vi "SizeGraphPanel.vi"(8 "ErrorIn(No Error)":errorcluster caption="entrée d'erreur (pas d'erreur)", 9 "Width Divider":i32, 10 "Height Divider":i32, 11 "PanRef":refnum<vi>) -> (0 "sortie d'erreur":errorcluster, 2 "Position":T1, 3 "cluster de sortie":T2 caption="Taille")   [LabVIEW 2010]
uses:
  <vilib>/Utility/miscctls.llb/LVBoundsTypeDef.ctl
  <vilib>/Utility/miscctls.llb/LVPositionTypeDef.ctl
  System.Windows.Forms
  System.Drawing
  <vilib>/Utility/miscctls.llb/LVPointTypeDef.ctl
panel:
  out "UpdtHorizLim":bool
  out "UpdtVertLim":bool
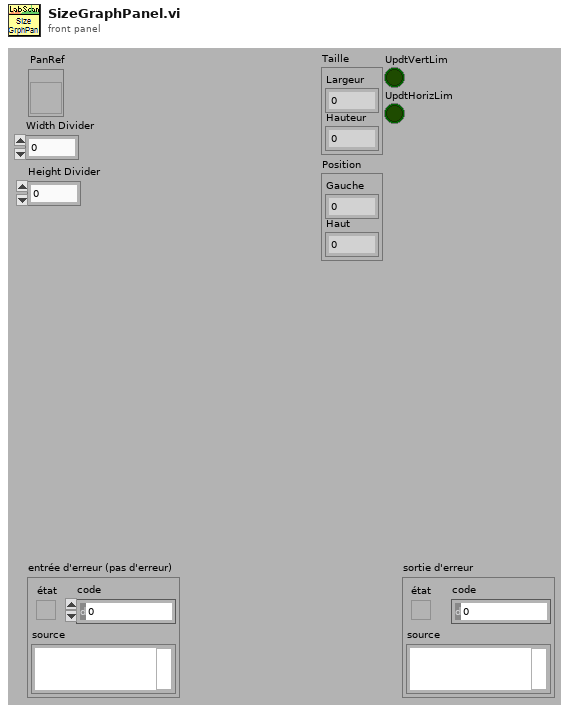
[diagram p1: front panel]
types:
  T1 = typedef "LVPositionTypeDef.ctl" = cluster{"Left":i32, "Top":i32}
  T2 = typedef "LVBoundsTypeDef.ctl" = cluster{"Width":u32, "Height":u32}
  T3 = enum32{"Invalid", "Standard", "Closed", "Hidden", "Minimized", "Maximized"}
  T4 = enum16{"Always On", "Always Off", "Off While Running"}
  T5 = typedef "LVPointTypeDef.ctl" = cluster{"Horizontal":i16, "Vertical":i16}
  T6 = typedef "LVRectTypeDef.ctl" = cluster{"left":i16, "top":i16, "right":i16, "bottom":i16}
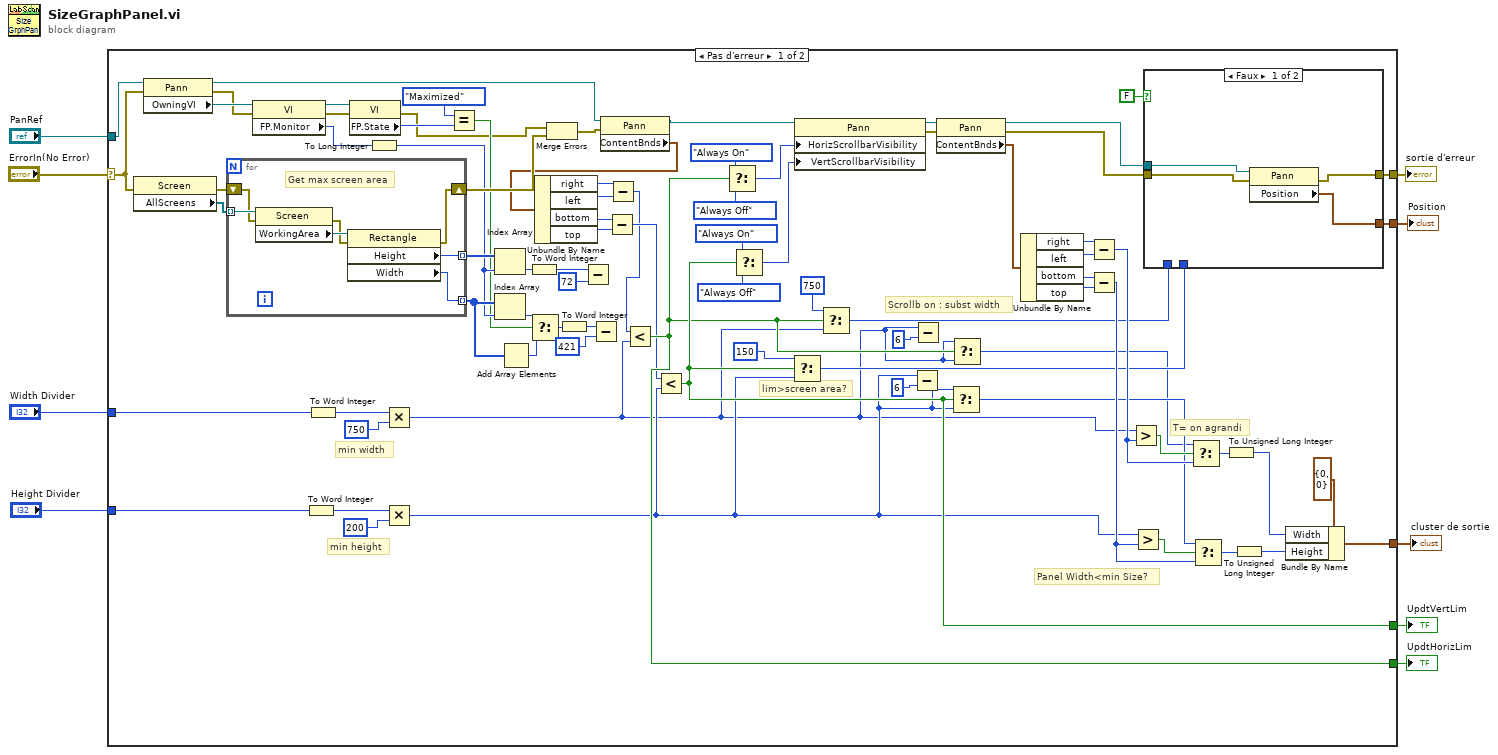
[diagram p0: block diagram]
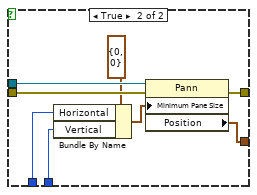
[diagram p2: hidden frame]
diagram:
  n1 = case shown="Pas d'erreur" "ErrorIn(No Error)" {
    selector: "ErrorIn(No Error)" -> [w58 w110]
    tunnel: [w86 w110] -> w8
    tunnel: "PanRef" -> [w59 _]
    tunnel: "Width Divider" -> [w90 _]
    tunnel: "Height Divider" -> [w84 _]
    tunnel: [w68 _] -> w4
    tunnel: [w81 _] -> w3
    tunnel: [w26 _] -> w2
    tunnel: [w25 _] -> w1
    frame No Error {
      # "min width"
      # "min height"
      # "Scrollb on : subst width"
      # "T= on agrandi"
      # "lim>screen area?"
      # "Panel Width<min Size?"
      n2 = property class="Screen"(error in=w58) -> (error out=w61:errorcluster, "AllScreens"=w64:refnum<k24>[])  [unwired: 1 in, 1 out]
      n3 = property class="Pann"(reference=w59, error in=w58) -> (reference out=w18:refnum<vi>, error out=w33:errorcluster, "OwningVI"=w63:refnum<vi>)
      n4 = for {
        tunnel: [w107] -> w54 mode=indexing
        tunnel: [w106] -> w62 mode=indexing
        tunnel: w64 -> [w104] mode=indexing
        shift-right: [w105] -> w67
        shift-left: w61 -> [w103]
        # "Get max screen area"
        n5 = property class="Screen"(reference=w104, error in=w103) -> (error out=w108:errorcluster, "WorkingArea"=w109:refnum<k24>)  [unwired: 1 out]
        n6 = property class="Rectangle"(reference=w109, error in=w108) -> (error out=w105:errorcluster, "Height"=w106:i32, "Width"=w107:i32)  [unwired: 1 out]
      }
      n7 = property class="VI"(reference=w63, error in=w33) -> (reference out=w32:refnum<vi>, error out=w28:errorcluster, "FP.Monitor"=w60:u16)
      n8 = To Word Integer(number=w84) -> (16bit integer=w82:i16)
      n9 = To Word Integer(number=w90) -> (16bit integer=w83:i16)
      n10 = property class="VI"(reference=w32, error in=w28) -> (error out=w27:errorcluster, "FP.State"=w30:T3)  [unwired: 1 out]
      n11 = To Long Integer(number=w60) -> (32bit integer=w53:i32)
      n12 = Multiply(x=w83, y=i16 750) -> (x*y=w21:i16)
      n13 = Multiply(x=w82, y=i16 200) -> (x*y=w22:i16)
      n14 = Equal?(x=T3."Maximized" ("Fenêtre face-avant : état"), y=w30) -> (x = y?=w29:bool)
      n15 = Index Array(array=w62, index=w53) -> (element=w56:i32)
      n16 = Index Array(array=w54, index=w53) -> (element=w52:i32)
      n17 = Add Array Elements(numeric array=w54) -> (sum=w51:i32)
      n18 = To Word Integer(number=w56) -> (16bit integer=w41:i16)
      n19 = Select(t=w52, s=w29, f=w51) -> (s? t:f=w50:i32)
      n20 = Merge Errors(w27, w67) -> (w19:errorcluster)
      n21 = To Word Integer(number=w50) -> (16bit integer=w40:i16)
      n22 = Subtract(x=w41, y=i16 72) -> ()  [unwired: 1 out]
      n23 = Subtract(x=w40, y=i16 421) -> ()  [unwired: 1 out]
      n24 = property class="Pann"(reference=w18, error in=w19) -> (reference out=w17:refnum<vi>, "ContentBnds"=w12:T6)  [unwired: 1 out]
      n25 = Unbundle By Name(w12) -> ("right"=w13:i16, "left"=w14:i16, "bottom"=w16:i16, "top"=w15:i16)
      n26 = Subtract(x=w16, y=w15) -> (x-y=w11:i16)
      n27 = Subtract(x=w13, y=w14) -> (x-y=w10:i16)
      n28 = Less?(x=w10, y=w21) -> (x < y?=w25:bool)
      n29 = Less?(x=w11, y=w22) -> (x < y?=w26:bool)
      n30 = Select(t=T4."Always On" ("Visibilité de la barre de défilement horizontale"), s=w25, f=T4."Always Off" ("Visibilité de la barre de défilement horizontale")) -> (s? t:f=w47:T4)
      n31 = Select(t=T4."Always On" ("Visibilité de la barre de défilement horizontale"), s=w26, f=T4."Always Off" ("Visibilité de la barre de défilement horizontale")) -> (s? t:f=w44:T4)
      n32 = Select(t=i16 150, s=w26, f=w22) -> (s? t:f=w36:i16)
      n33 = property class="Pann"(reference=w17, "HorizScrollbarVisibility"=w47, "VertScrollbarVisibility"=w44) -> (reference out=w66:refnum<vi>, error out=w65:errorcluster)  [unwired: 1 in]
      n34 = Select(t=i16 750, s=w25, f=w21) -> (s? t:f=w37:i16)
      n35 = Subtract(x=w22, y=i16 6) -> ()  [unwired: 1 out]
      n36 = Subtract(x=w21, y=i16 6) -> ()  [unwired: 1 out]
      n37 = property class="Pann"(reference=w66, error in=w65) -> (reference out=w88:refnum<vi>, error out=w87:errorcluster, "ContentBnds"=w77:T6)
      n38 = Select(t=w22, s=w26, f=w22) -> (s? t:f=w35:i16)
      n39 = Select(t=w21, s=w25, f=w21) -> (s? t:f=w34:i16)
      n40 = Unbundle By Name(w77) -> ("right"=w76:i16, "left"=w75:i16, "bottom"=w73:i16, "top"=w74:i16)
      n41 = Subtract(x=w76, y=w75) -> (x-y=w43:i16)
      n42 = Subtract(x=w73, y=w74) -> (x-y=w42:i16)
      n43 = Greater?(x=w21, y=w43) -> (0:w80:bool)
      n44 = Greater?(x=w22, y=w42) -> (0:w79:bool)
      n45 = case shown="Faux" FALSE {
        tunnel: w88 -> [w93 w102]
        tunnel: w87 -> [w92 w101]
        tunnel: [w91 w100] -> w86
        tunnel: [w94 w99] -> w68
        tunnel: w37 -> [_ w98]
        tunnel: w36 -> [_ w97]
        frame False {
          n46 = property class="Pann"(reference=w93, error in=w92) -> (error out=w91:errorcluster, "Position"=w94:T1)  [unwired: 1 out]
        }
        frame True {
          n47 = Bundle By Name(cluster=T5 {"Horizontal"=0, "Vertical"=0} ("Taille minimale de panneau"), "Horizontal"=w98, "Vertical"=w97) -> (w95:T5)
          n48 = property class="Pann"(reference=w102, error in=w101, "Minimum Pane Size"=w95) -> (error out=w100:errorcluster, "Position"=w99:T1)  [unwired: 1 out]
        }
      }
      n49 = Select(t=w34, s=w80, f=w43) -> (s? t:f=w71:i16)
      n50 = Select(t=w35, s=w79, f=w42) -> (s? t:f=w78:i16)
      n51 = To Unsigned Long Integer(number=w71) -> (unsigned 32bit integer=w70:u32)
      n52 = To Unsigned Long Integer(number=w78) -> (unsigned 32bit integer=w69:u32)
      n53 = Bundle By Name(cluster=T2 {"Width"=0, "Height"=0} ("cluster de sortie"), "Width"=w70, "Height"=w69) -> (w81:T2)
    }
    frame Error {
    }
  }
  "sortie d'erreur" <- w8
  "cluster de sortie" <- w3
  "Position" <- w4
  "UpdtVertLim" <- w2
  "UpdtHorizLim" <- w1
